vi "Main.vi"() -> ()   [LabVIEW 2019]
doc: "This Continuous Measurement sample project is based on the Queued Message Handler template.\n\nThe Event Handling Loop generates messages based on user interface actions.\n\nThe Message Handling Loop processes messages generated by the Event Handling Loop, or by other messages. There are also Acquisition and Logging message handling loop subVIs, and a chart updating loop."
uses:
  Controls/Acquired Data.ctl
  Settings/Settings.ctl
  Acquisition/Hardware Configuration.ctl
  Acquisition/Signal Type.ctl
  Logging/Logging Configuration.ctl
  Controls/UI State.ctl
  Support/Message Queue/Enqueue Message (Single).vi
  Support/Message Queue/Enqueue Message (Array).vi
  <vilib>/Utility/error.llb/Error Cluster From Error Code.vi
  <vilib>/ErrorRing/Error Ring.xnode
  Acquisition/Acquisition.lvlib
  Logging/Logging.lvlib
  Settings/Settings.lvlib
  Support/User Event - Stop/User Event - Stop.lvlib
  Support/Message Queue/Message Queue.lvlib
  Settings/Settings Dialog.vi
panel:
  in  "Data":T1
  out "User Event - Stop":refnum<user-event>
  out "Data":T1(graph)
  in  "Settings":bool
  in  "Start":bool
  in  "Stop":bool
  out "Status":string
  in  "Exit":bool
  # "Continuous Measurement Data Logger"
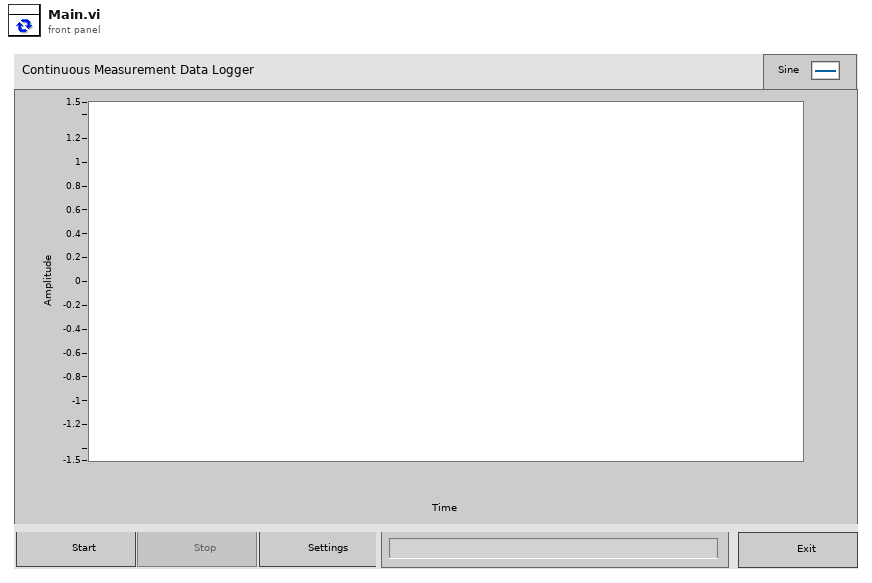
[diagram p1: front panel]
types:
  T1 = typedef "Acquired Data.ctl" = waveform(dbl)[]
  T2 = typedef "UI State.ctl" = enum16{"Idle", "Acquiring and Logging", "Waiting for Exit", "Waiting for Exit (Acq Stopped)", "Waiting for Exit (Log Stopped)", "Waiting for Stop", "Waiting for Stop (Acq Stopped)", "Waiting for Stop (Log Stopped)"}
  T3 = typedef "Settings.lvlib/Settings.ctl" = cluster{"Hardware Configuration":T4, "Logging Configuration":T6, "UI Refs":cluster{"Start Ref":refnum<vi>, "Settings Ref":refnum<vi>, "Stop Ref":refnum<vi>, "Exit Ref":refnum<vi>, "Status Ref":refnum<vi>, "Data Ref":refnum<vi>}}
  T4 = typedef "Acquisition.lvlib/Hardware Configuration.ctl" = cluster{"HW Refnum <Replace Me>":string, "Signal Type <Replace Me>":T5}
  T5 = typedef "Acquisition.lvlib/Signal Type.ctl" = enum16{"Sine Wave", "Square with Noise"}
  T6 = typedef "Logging.lvlib/Logging Configuration.ctl" = cluster{"Log File Base Path":path, "TDMS File Reference":refnum<k34>}
  T7 = typedef "Message Queue.lvlib/All Message Queues.ctl" = cluster{"Message Queues":cluster{"UI":refnum<queue>, "Acquisition":refnum<queue>, "Logging":refnum<queue>}, "Data Queues & Notifier":cluster{"Data Queue":T8, "Data Notifer":T9}}
  T8 = typedef "Data Queue.ctl" = refnum<queue>
  T9 = typedef "Data Notifier.ctl" = refnum<notifier>
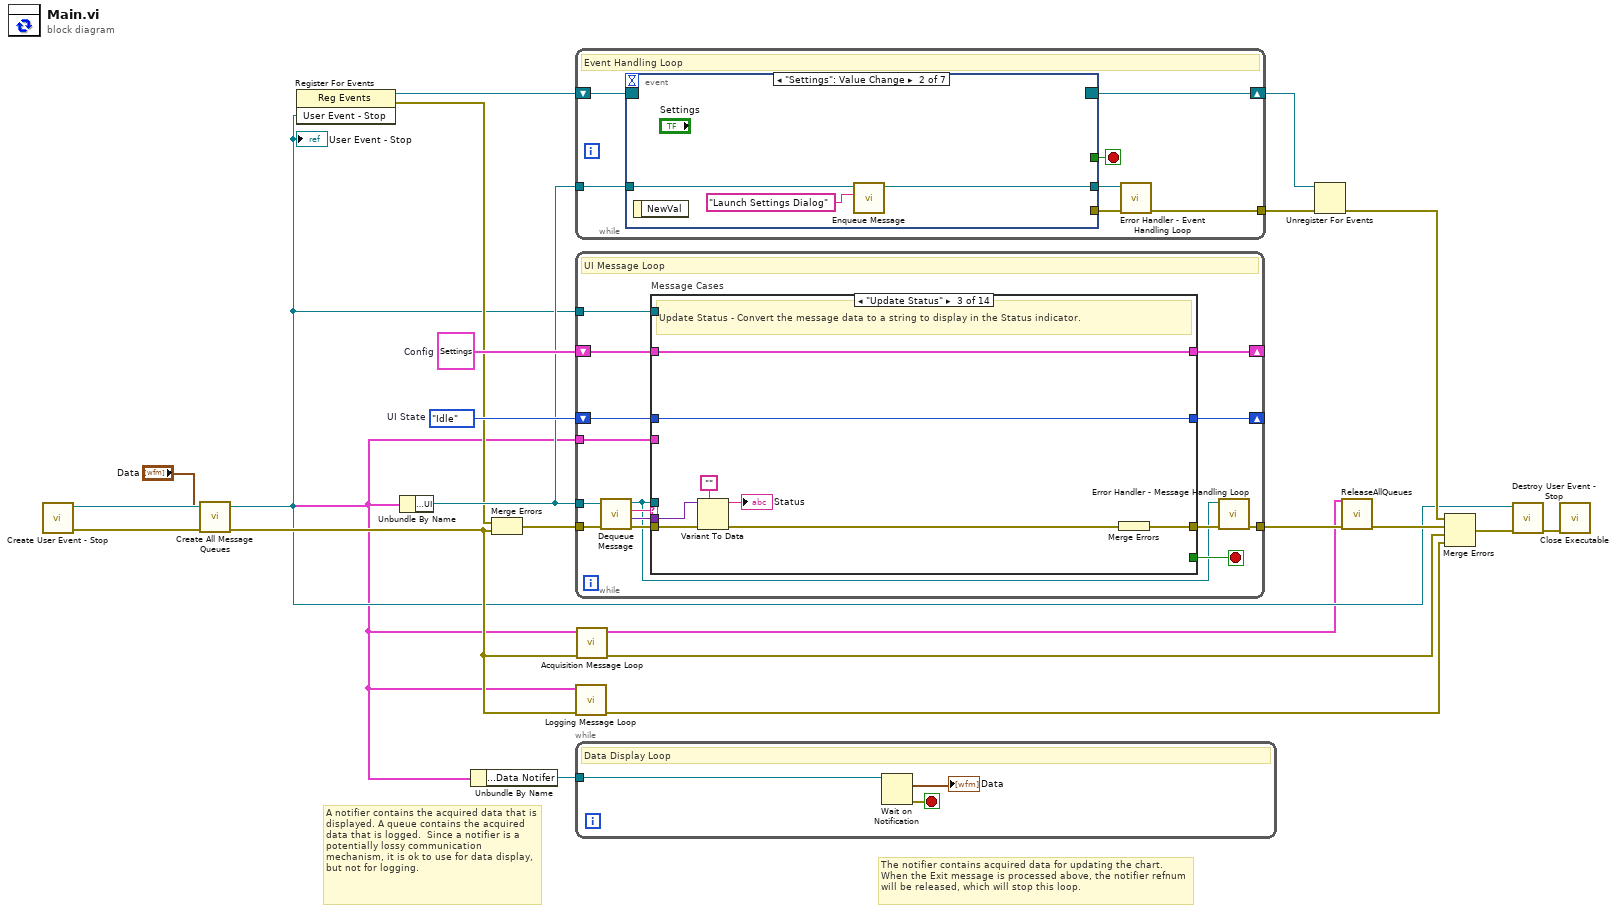
[diagram p0: block diagram]
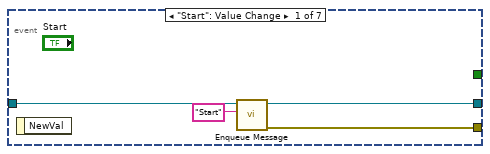
[diagram p2: hidden frame]
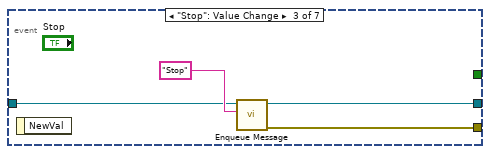
[diagram p3: hidden frame]
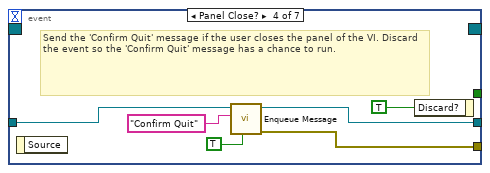
[diagram p4: hidden frame]
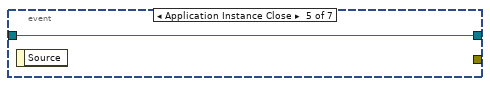
[diagram p5: hidden frame]
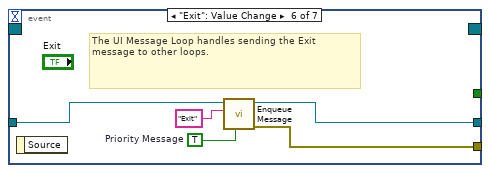
[diagram p6: hidden frame]
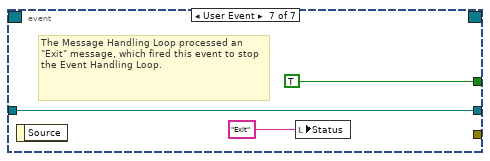
[diagram p7: hidden frame]
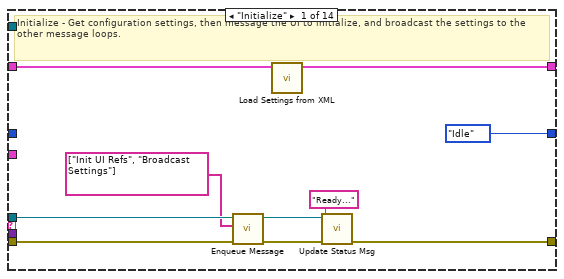
[diagram p8: hidden frame]
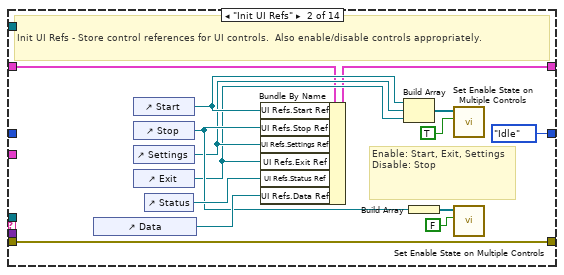
[diagram p9: hidden frame]
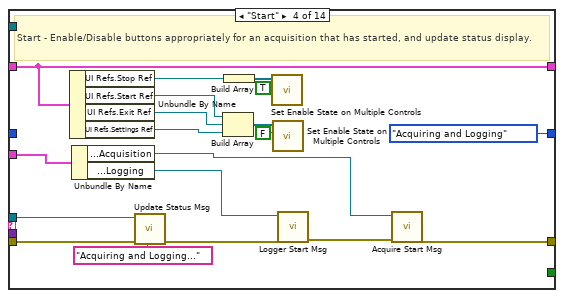
[diagram p10: hidden frame]
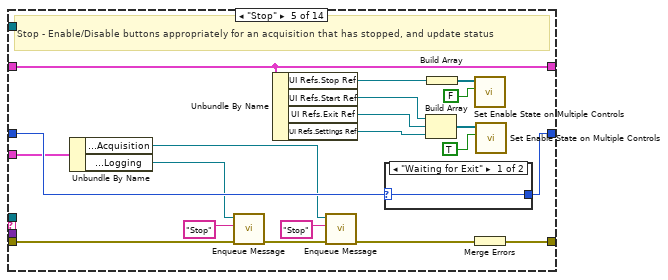
[diagram p11: hidden frame]
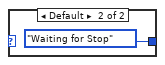
[diagram p12: hidden frame]
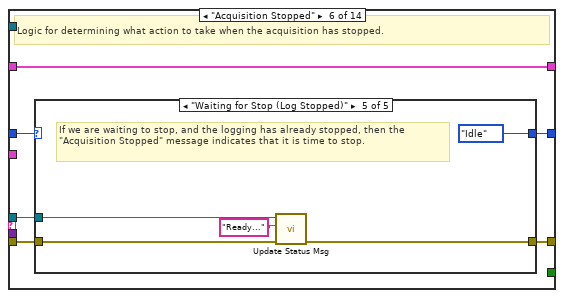
[diagram p13: hidden frame]
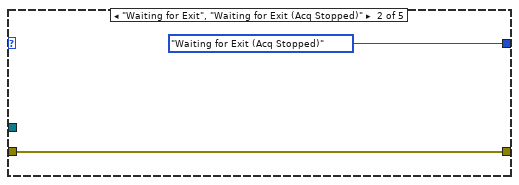
[diagram p15: hidden frame]
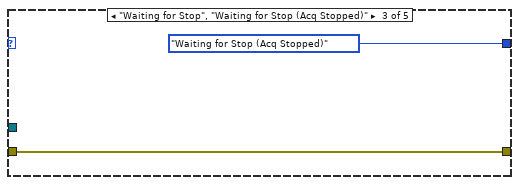
[diagram p16: hidden frame]
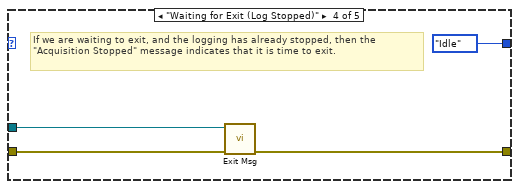
[diagram p17: hidden frame]
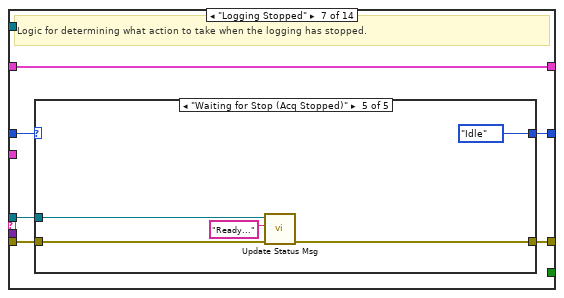
[diagram p18: hidden frame]
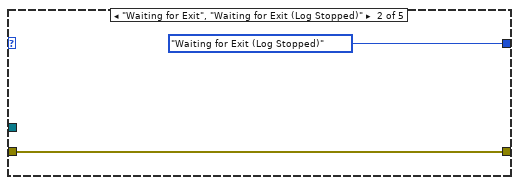
[diagram p20: hidden frame]
diagram:
  w12 = UI_State."Idle"  # UI State
  w15 = T3 {"Hardware Configuration"={"HW Refnum <Replace Me>"="", "Signal Type <Replace Me>"=enum."Sine Wave"}, "Logging Configuration"={"Log File Base Path"=path "", "TDMS File Reference"=refnum}, "UI Refs"={"Start Ref"=refnum, "Settings Ref"=refnum, "Stop Ref"=refnum, "Exit Ref"=refnum, "Status Ref"=refnum, "Data Ref"=refnum}}  # Config
  # "A notifier contains the acquired data that is displayed. A queue contains the acquired data that is logged.  Since a notifier is a potentially lossy communication mechanism, it is ok to use for data display, but not for logging."
  # "The notifier contains acquired data for updating the chart. When the Exit message is processed above, the notifier refnum will be released, which will stop this loop."
  n1 = call "Create User Event - Stop.vi"() -> ("error out"=w18:errorcluster, "User Event - Stop"=w4:refnum<user-event>)  [unwired: 10 in]
  "User Event - Stop" <- w4
  n2 = call "Create All Message Queues.vi"("error in (no error)"=w18, "Data"="Data") -> ("error out"=w16:errorcluster, "Message Queues out"=w1:T7)  [unwired: 8 in]
  n3 = register-events(w4) -> (reference out=w7:refnum<event-registration>, error out=w5:errorcluster)  [unwired: 2 in]
  n4 = Unbundle By Name(w1) -> ("Message Queues.UI"=w10:refnum<queue>)
  n5 = Unbundle By Name(w1) -> ("Data Queues & Notifier.Data Notifer"=w3:T9)
  n6 = Merge Errors(w5, w16) -> (w6:errorcluster)
  n7 = while {
    tunnel: w10 -> [w27]
    tunnel: [w24] -> w20
    shift-right: [w26] -> w13
    shift-left: w7 -> [w28]
    stop <- w25 stop-if-true
    # "Event Handling Loop"
    n8 = event shown="[1] \"Settings\": Value Change" {
      selector: w28 -> [_ _ _ _ _ _ _]
      dyn-events: [_ _ _ _ _ _ _] -> w26
      timeout: _ -> [_ _ _ _ _ _ _]
      tunnel: [_ _ _ _ _ _ TRUE ("Discard?")] -> w25
      tunnel: w27 -> [w32 w34 w38 w43 w46 w48 w52]
      tunnel: [w30 _ w37 w41 _ w51 _] -> w23
      tunnel: [w29 w33 w36 w42 w46 w47 w52] -> w22
      event "Start": Value Change {
        n9 = event-data() -> ()  [unwired: 1 in, 1 out]
        n10 = call-poly "Enqueue Message.vi"("Message"="Start", "Message Queue"=w32) -> ("error out"=w30:errorcluster, "dup Message Queue"=w29:refnum<queue>)  [unwired: 8 in]
      }
      event "Settings": Value Change {
        n11 = event-data() -> ()  [unwired: 1 in, 1 out]
        n12 = call-poly "Enqueue Message.vi"("Message"="Launch Settings Dialog", "Message Queue"=w34) -> ("dup Message Queue"=w33:refnum<queue>)  [unwired: 8 in, 1 out]
      }
      event "Stop": Value Change {
        n13 = event-data() -> ()  [unwired: 1 in, 1 out]
        n14 = call-poly "Enqueue Message.vi"("Message"="Stop", "Message Queue"=w38) -> ("error out"=w37:errorcluster, "dup Message Queue"=w36:refnum<queue>)  [unwired: 8 in]
      }
      event Panel Close? {
        # "Send the 'Confirm Quit' message if the user closes the panel of the VI. Discard the event so the 'Confirm Quit' message has a chance to run."
        n15 = event-data() -> ()  [unwired: 1 in, 1 out]
        n16 = call-poly "Enqueue Message.vi"("Priority Message? (F)"=TRUE, "Message"="Confirm Quit", "Message Queue"=w43) -> ("error out"=w41:errorcluster, "dup Message Queue"=w42:refnum<queue>)  [unwired: 7 in]
        n17 = event-data("Discard?"=TRUE) -> ()  [unwired: 1 in, 1 out]
      }
      event Application Instance Close {
        n18 = event-data() -> ()  [unwired: 1 in, 1 out]
      }
      event "Exit": Value Change {
        w49 = TRUE  # Priority Message
        # "The UI Message Loop handles sending the Exit message to other loops."
        n19 = event-data() -> ()  [unwired: 1 in, 1 out]
        n20 = call-poly "Enqueue Message.vi"("Priority Message? (F)"=w49, "Message"="Exit", "Message Queue"=w48) -> ("error out"=w51:errorcluster, "dup Message Queue"=w47:refnum<queue>)  [unwired: 7 in]
      }
      event User Event {
        # "The Message Handling Loop processed an \"Exit\" message, which fired this event to stop the Event Handling Loop."
        n21 = event-data() -> ()  [unwired: 1 in, 1 out]
        n22 = local write "Status"("Exit" ("Exit String")) -> ()
      }
    }
    n23 = call "Error Handler - Event Handling Loop.vi"("error in (no error)"=w23, "Message Queue"=w22) -> ("dup error in"=w24:errorcluster)  [unwired: 8 in, 1 out]
  }
  n24 = while {
    tunnel: w10 -> [w63]
    tunnel: w4 -> [w68]
    shift-right: [w62] -> _
    shift-left: w15 -> [w61]
    shift-right: [w56] -> _
    shift-left: w12 -> [w57]
    tunnel: w6 -> [w67]
    tunnel: [w60] -> w21
    tunnel: w1 -> [w55]
    stop <- w69 stop-if-true
    # "UI Message Loop"
    n25 = call "Dequeue Message.vi"("error in (no error)"=w67, "Message Queue"=w63) -> ("error out"=w66:errorcluster, "Message Data"=w64:variant, "Message"=w65:string, "dup Message Queue"=w58:refnum<queue>)  [unwired: 6 in]
    n26 = case "Message Cases" shown="\"Update Status\"" w65 {
      selector: w65 -> [_ _ _ _ _ _ _ _ _ _ _ _ _ w265]
      tunnel: w58 -> [w77 _ _ w105 _ w145 w166 _ w201 _ w220 _ _ _]
      tunnel: w66 -> [w76 w93 w100 w104 w139 w146 w167 w190 w203 w209 w219 w250 w263 _]
      tunnel: [w70 w93 w101 w111 w140 w143 w164 w196 w197 w212 w218 w257 w262 w264] -> w59
      tunnel: [_ _ _ _ _ _ _ _ _ _ _ TRUE _ _] -> w69
      tunnel: w64 -> [_ _ w99 _ _ _ _ _ _ w213 _ w248 _ _]
      tunnel: w68 -> [_ _ _ _ _ _ _ _ _ _ _ w258 _ _]
      tunnel: [w78 w80 w95 w109 w124 w148 w169 w194 w200 w216 w222 w256 w261 w267] -> w62
      tunnel: w61 -> [w79 w81 w95 w109 w124 w148 w169 w194 w204 w216 w222 w256 w261 w267]
      tunnel: w57 -> [_ _ w94 _ w125 w147 w168 w188 w198 w211 w221 _ w260 w266]
      tunnel: [UI_State."Idle" ("UI State") UI_State."Idle" ("UI State") w94 UI_State."Acquiring and Logging" ("UI State") w126 w144 w165 w188 w198 w211 w217 UI_State."Idle" ("UI State") w260 w266] -> w56
      tunnel: w55 -> [_ _ _ w108 w123 _ _ w187 _ _ _ w246 _ _]
      frame "Initialize" {
        # "Initialize - Get configuration settings, then message the UI to initialize, and broadcast the settings to the other message loops."
        n27 = call-poly "Enqueue Message.vi"("error in (no error)"=w76, "Message Array"=string[] ["Init UI Refs", "Broadcast Settings"], "Message Queue"=w77) -> ("error out"=w71:errorcluster, "dup Message Queue"=w73:refnum<queue>)  [unwired: 7 in]
        n28 = call "Load Settings from XML.vi"("Settings in"=w79) -> ("Settings out"=w78:T3)  [unwired: 9 in, 1 out]
        n29 = call "Update Status Msg.vi"("error in (no error)"=w71, "Ready..."="Ready...", "Queue in"=w73) -> ("error out"=w70:errorcluster)  [unwired: 8 in]
      }
      frame "Init UI Refs" {
        # "Enable: Start, Exit, Settings\nDisable: Stop"
        # "Init UI Refs - Store control references for UI controls.  Also enable/disable controls appropriately."
        n30 = control-ref of="Data"() -> (w91:refnum<vi>)
        n31 = control-ref of="Start"() -> (w85:refnum<vi>)
        n32 = control-ref of="Stop"() -> (w86:refnum<vi>)
        n33 = control-ref of="Settings"() -> (w84:refnum<vi>)
        n34 = control-ref of="Exit"() -> (w83:refnum<vi>)
        n35 = control-ref of="Status"() -> (w92:refnum<vi>)
        n36 = Bundle By Name(cluster=w81, "UI Refs.Start Ref"=w85, "UI Refs.Stop Ref"=w86, "UI Refs.Settings Ref"=w84, "UI Refs.Exit Ref"=w83, "UI Refs.Status Ref"=w92, "UI Refs.Data Ref"=w91) -> (w80:T3)
        n37 = Build Array(w85, w84, w83) -> (w89:refnum<vi>[])
        n38 = Build Array(w86) -> (w88:refnum<vi>[])
        n39 = call "Set Enable State on Multiple Controls.vi"("Enable?"=TRUE, "Controls"=w89) -> ()  [unwired: 10 in]
        n40 = call "Set Enable State on Multiple Controls.vi"("Enable?"=FALSE, "Controls"=w88) -> ()  [unwired: 10 in]
      }
      frame "Update Status" {
        # "Update Status - Convert the message data to a string to display in the Status indicator."
        n41 = Variant To Data(error in=w100, type="", Variant=w99) -> (data=→"Status":string, error out=w97:errorcluster)
        n42 = Merge Errors(w97) -> (w101:errorcluster)
      }
      frame "Start" {
        # "Start - Enable/Disable buttons appropriately for an acquisition that has started, and update status display."
        n43 = Unbundle By Name(w109) -> ("UI Refs.Stop Ref"=w116:refnum<vi>, "UI Refs.Start Ref"=w115:refnum<vi>, "UI Refs.Exit Ref"=w114:refnum<vi>, "UI Refs.Settings Ref"=w113:refnum<vi>)
        n44 = Unbundle By Name(w108) -> ("Message Queues.Acquisition"=w107:refnum<queue>, "Message Queues.Logging"=w106:refnum<queue>)
        n45 = call "Update Status Msg.vi"("error in (no error)"=w104, "Ready..."="Acquiring and Logging..." ("Acquiring and Logging..."), "Queue in"=w105) -> ("error out"=w103:errorcluster)  [unwired: 8 in]
        n46 = Build Array(w115, w114, w113) -> (w119:refnum<vi>[])
        n47 = Build Array(w116) -> (w118:refnum<vi>[])
        n48 = call "Set Enable State on Multiple Controls.vi"("Enable?"=TRUE, "Controls"=w118) -> ()  [unwired: 10 in]
        n49 = call "Set Enable State on Multiple Controls.vi"("Enable?"=FALSE, "Controls"=w119) -> ()  [unwired: 10 in]
        n50 = call "Logger Start Msg.vi"("error in (no error)"=w103, "Queue in"=w106) -> ("error out"=w112:errorcluster)  [unwired: 9 in]
        n51 = call "Acquire Start Msg.vi"("error in (no error)"=w112, "Queue in"=w107) -> ("error out"=w111:errorcluster)  [unwired: 9 in]
      }
      frame "Stop" {
        # "Stop - Enable/Disable buttons appropriately for an acquisition that has stopped, and update status"
        n52 = Unbundle By Name(w123) -> ("Message Queues.Acquisition"=w122:refnum<queue>, "Message Queues.Logging"=w121:refnum<queue>)
        n53 = call-poly "Enqueue Message.vi"("error in (no error)"=w139, "Message"="Stop", "Message Queue"=w121) -> ("error out"=w129:errorcluster)  [unwired: 7 in, 1 out]
        n54 = Unbundle By Name(w124) -> ("UI Refs.Stop Ref"=w134:refnum<vi>, "UI Refs.Start Ref"=w133:refnum<vi>, "UI Refs.Exit Ref"=w132:refnum<vi>, "UI Refs.Settings Ref"=w131:refnum<vi>)
        n55 = call-poly "Enqueue Message.vi"("error in (no error)"=w129, "Message"="Stop", "Message Queue"=w122) -> ("error out"=w128:errorcluster)  [unwired: 7 in, 1 out]
        n56 = case shown="\"Waiting for Exit\"" w125 {
          selector: w125 -> [w141 _]
          tunnel: [w141 UI_State."Waiting for Stop" ("UI State")] -> w126
          frame "Waiting for Exit" {
          }
          frame Default {
          }
        }
        n57 = Build Array(w133, w132, w131) -> (w137:refnum<vi>[])
        n58 = Build Array(w134) -> (w136:refnum<vi>[])
        n59 = call "Set Enable State on Multiple Controls.vi"("Enable?"=FALSE, "Controls"=w136) -> ()  [unwired: 10 in]
        n60 = Merge Errors(w128) -> (w140:errorcluster)
        n61 = call "Set Enable State on Multiple Controls.vi"("Enable?"=TRUE, "Controls"=w137) -> ()  [unwired: 10 in]
      }
      frame "Acquisition Stopped" {
        # "Logic for determining what action to take when the acquisition has stopped."
        n62 = case shown="\"Waiting for Stop (Log Stopped)\"" w147 {
          selector: w147 -> [w150 _ _ _ _]
          tunnel: w146 -> [w149 w152 w154 w157 w161]
          tunnel: w145 -> [_ _ _ w156 w162]
          tunnel: [w150 UI_State."Waiting for Exit (Acq Stopped)" ("UI State") UI_State."Waiting for Stop (Acq Stopped)" ("UI State") UI_State."Idle" ("UI State") UI_State."Idle" ("UI State")] -> w144
          tunnel: [w149 w152 w154 w155 w160] -> w143
          frame Default {
          }
          frame "Waiting for Exit", "Waiting for Exit (Acq Stopped)" {
          }
          frame "Waiting for Stop", "Waiting for Stop (Acq Stopped)" {
          }
          frame "Waiting for Exit (Log Stopped)" {
            # "If we are waiting to exit, and the logging has already stopped, then the \"Acquisition Stopped\" message indicates that it is time to exit."
            n63 = call "Exit Msg.vi"("error in (no error)"=w157, "Queue in"=w156) -> ("error out"=w155:errorcluster)  [unwired: 9 in]
          }
          frame "Waiting for Stop (Log Stopped)" {
            # "If we are waiting to stop, and the logging has already stopped, then the \"Acquisition Stopped\" message indicates that it is time to stop."
            n64 = call "Update Status Msg.vi"("error in (no error)"=w161, "Ready..."="Ready...", "Queue in"=w162) -> ("error out"=w160:errorcluster)  [unwired: 8 in]
          }
        }
      }
      frame "Logging Stopped" {
        # "Logic for determining what action to take when the logging has stopped."
        n65 = case shown="\"Waiting for Stop (Acq Stopped)\"" w168 {
          selector: w168 -> [w171 _ _ _ _]
          tunnel: w167 -> [w170 w173 w175 w179 w182]
          tunnel: w166 -> [_ _ _ w177 w181]
          tunnel: [w171 UI_State."Waiting for Exit (Log Stopped)" ("UI State") UI_State."Waiting for Stop (Log Stopped)" ("UI State") UI_State."Idle" ("UI State") UI_State."Idle" ("UI State")] -> w165
          tunnel: [w170 w173 w175 w178 w180] -> w164
          frame Default {
          }
          frame "Waiting for Exit", "Waiting for Exit (Log Stopped)" {
          }
          frame "Waiting for Stop", "Waiting for Stop (Log Stopped)" {
          }
          frame "Waiting for Exit (Acq Stopped)" {
            n66 = call "Exit Msg.vi"("error in (no error)"=w179, "Queue in"=w177) -> ("error out"=w178:errorcluster)  [unwired: 9 in]
          }
          frame "Waiting for Stop (Acq Stopped)" {
            n67 = call "Update Status Msg.vi"("error in (no error)"=w182, "Ready..."="Ready...", "Queue in"=w181) -> ("error out"=w180:errorcluster)  [unwired: 8 in]
          }
        }
      }
      frame "Broadcast settings" {
        w189 = "Update Settings" ("Message")
        # "Broadcast settings - Send the 'Update Settings' message to the Logging and Acquisition message loops."
        n68 = Unbundle By Name(w194) -> ("Hardware Configuration"=w193:T4, "Logging Configuration"=w192:T6)
        n69 = Unbundle By Name(w187) -> ("Message Queues.Acquisition"=w186:refnum<queue>, "Message Queues.Logging"=w185:refnum<queue>)
        n70 = call-poly "Enqueue Message.vi"("Message Data"=w193, "Message"=w189, "Message Queue"=w186) -> ("error out"=w195:errorcluster)  [unwired: 7 in, 1 out]
        n71 = call-poly "Enqueue Message.vi"("error in (no error)"=w195, "Message Data"=w192, "Message"=w189, "Message Queue"=w185) -> ("error out"=w191:errorcluster)  [unwired: 6 in, 1 out]
        n72 = Merge Errors(w191, w190) -> (w196:errorcluster)
      }
      frame "Launch Settings Dialog" {
        # "Launch Settings Dialog - Launch the Settings Dialog when the user clicks the 'Settings' button."
        n73 = call-by-ref "?"("error in (no error)"=w203, "Settings in"=w204) -> ("error out"=w199:errorcluster, "Cancelled?"=w202:bool, "Settings out"=w200:T3)  [unwired: 8 in, 3 out]
        n74 = case shown="False" w202 {
          tunnel: w201 -> [w207 _]
          tunnel: w199 -> [w206 w208]
          tunnel: [w205 w208] -> w197
          frame False {
            n75 = call "Broadcast Settings Msg.vi"("error in (no error)"=w206, "Queue in"=w207) -> ("error out"=w205:errorcluster)  [unwired: 9 in]
          }
          frame True {
          }
        }
      }
      frame "Error" {
        # "Error - Display an error dialog. This message is sent by the \"Error Handler\" VIs at the end of other loops in this application."
        n76 = Variant To Data(error in=w209, type=errorcluster {"status"=FALSE, "code"=0, "source"=""} ("error constant"), Variant=w213) -> (data=w210:errorcluster, error out=w214:errorcluster)
        n77 = call <vilib>:"Simple Error Handler.vi"("error in (no error)"=w210) -> ()  [unwired: 4 in, 5 out]
        n78 = Merge Errors(w214) -> (w212:errorcluster)
      }
      frame "Confirm Quit" {
        # "Confirm Quit - Message that can confirm whether or not the user wants to exit the application."
        n79 = case shown="\"Acquiring and Logging\"" w221 {
          tunnel: w220 -> [w228 w232]
          tunnel: w219 -> [w227 w231]
          tunnel: [w226 w230] -> w218
          tunnel: [UI_State."Idle" ("UI State") w229] -> w217
          frame Default {
            # "If 'Confirm Quit' comes in while the system is idle, there is no need for a confirmation message."
            n80 = call-poly "Enqueue Message.vi"("Priority Message? (F)"=TRUE, "error in (no error)"=w227, "Message"="Exit", "Message Queue"=w228) -> ("error out"=w226:errorcluster)  [unwired: 6 in, 1 out]
          }
          frame "Acquiring and Logging" {
            n81 = Two Button Dialog(message="Are you sure you want to quit while the acquisition is running?" ("Confirm Quit Message"), 1:"No" ("No"), 2:"Yes" ("Yes")) -> (T button?=w233:bool)
            n82 = case shown="True" w233 {
              tunnel: w232 -> [_ w241]
              tunnel: w231 -> [w238 w242]
              tunnel: [w238 w240] -> w230
              tunnel: [UI_State."Acquiring and Logging" ("UI State") UI_State."Waiting for Exit" ("UI State")] -> w229
              frame False {
                # "User did not want to quit."
              }
              frame True {
                n83 = call "Stop Msg.vi"("error in (no error)"=w242, "Queue in"=w241) -> ("error out"=w240:errorcluster)  [unwired: 9 in]
              }
            }
          }
        }
      }
      frame "Exit" {
        w253 = "Exit" ("Message")
        # "Popup an error dialog if 'Exit' was called as a result of an error."
        # "Stop the VI"
        # "Exit - Send Exit messages to the Acquisition and Logging loops, and fire the user event to stop the Event Handling Loop."
        n84 = Unbundle By Name(w246) -> ("Message Queues.Acquisition"=w245:refnum<queue>, "Message Queues.Logging"=w244:refnum<queue>)
        n85 = Variant To Data(type=errorcluster {"status"=FALSE, "code"=0, "source"=""} ("error constant"), Variant=w248) -> (data=w247:errorcluster)  [unwired: 1 in, 1 out]
        n86 = call <vilib>:"Simple Error Handler.vi"("error in (no error)"=w247) -> ()  [unwired: 4 in, 5 out]
        n87 = call-poly "Enqueue Message.vi"("Priority Message? (F)"=TRUE, "error in (no error)"=w250, "Message"=w253, "Message Queue"=w245) -> ("error out"=w254:errorcluster)  [unwired: 6 in, 1 out]
        n88 = call-poly "Enqueue Message.vi"("Priority Message? (F)"=TRUE, "error in (no error)"=w254, "Message"=w253, "Message Queue"=w244) -> ("error out"=w251:errorcluster)  [unwired: 6 in, 1 out]
        n89 = call "Fire User Event - Stop.vi"("error in (no error)"=w251, "User Event - Stop"=w258) -> ("error out"=w257:errorcluster)  [unwired: 9 in]
      }
      frame "---Copy This Frame---" {
        # "Duplicate this frame when creating new messages.  Change this comment in the duplicated frame to describe this message."
        n90 = Merge Errors(w263) -> (w262:errorcluster)
      }
      frame Default {
        # "'Default' case only runs if there is a message that isn't defined in any of the other cases.  Output a programming error."
        n91 = xnode "Error Ring"("parameter 0"=w265) -> ("error out"=w264:errorcluster)
      }
    }
    n92 = call "Error Handler - Message Handling Loop.vi"("error in (no error)"=w59, "Message Queue"=w58) -> ("dup error in"=w60:errorcluster)  [unwired: 8 in, 1 out]
  }
  n93 = call "Logging Message Loop.vi"("error in (no error)"=w16, "Message Queues"=w1) -> ("error out"=w17:errorcluster)  [unwired: 9 in]
  n94 = while "Data Display Loop" {
    tunnel: w3 -> [w277]
    stop <- w276 stop-if-true
    # "Data Display Loop"
    n95 = Wait on Notification(notifier=w277) -> (notification=→"Data":T1, error out=w276:errorcluster)  [unwired: 3 in, 2 out]
  }
  n96 = call "Acquisition Message Loop.vi"("error in (no error)"=w16, "Message Queues"=w1) -> ("error out"=w19:errorcluster)  [unwired: 9 in]
  n97 = Unregister For Events(event registration refnum=w13, error in=w20) -> (error out=w14:errorcluster)
  n98 = call "ReleaseAllQueues.vi"("error in (no error)"=w21, "Message Queues"=w1) -> ("error out"=w8:errorcluster)  [unwired: 9 in]
  n99 = Merge Errors(w14, w8, w19, w17) -> (w11:errorcluster)
  n100 = call "Destroy User Event - Stop.vi"("error in (no error)"=w11, "User Event - Stop"=w4) -> ("error out"=w9:errorcluster)  [unwired: 9 in]
  n101 = call "Close Executable.vi"("error in (no error)"=w9) -> ()  [unwired: 11 in]
